vi "NN_Layer_Get_OutRefs_as3D_Tensor.vi"(8 "error in (no error)":errorcluster, 11 "Layer":T1={"Name"="", "Layer_Data"=variant, "Layer_Type"=enum."Input3D", "Dims_In"={"C"=0, "H"=0, "W"=0}, "Layers_In"=variant, "Dims_Out"={"C"=0, "H"=0, "W"=0}, "Layers_Out"=variant, "Metrics"={"Data"=0.0, "Params"=0.0, "Ops"=0.0}, "GPU_Data"=variant, "mBatch"=0, "NN_Device"=enum."CPU", "NNg_hdls"={"cudnn"=0, "cublas"=0, "stream"=0, "curand"=0}, "Train?"=FALSE, "Dimty"=enum."1D", "RecptField"={"Dims"={"V"=0, "H"=0}, "J"={"V"=0, "H"=0}}} {"Metrics"."Data" format="%#_4p"; "Metrics"."Params" format="%#_4p"; "Metrics"."Ops" format="%#_4p"}) -> (0 "error out":errorcluster, 2 "dOut":refnum<class "T4D_SGL.lvclass">, 3 "Out":refnum<class "T4D_SGL.lvclass">)   [LabVIEW 2020]
uses:
  <vilib>/Ngene/Deep Learning Toolkit/Toolkit/NN_Layers/Controls/NN_Layer.ctl
  <vilib>/Ngene/Deep Learning Toolkit/Toolkit/NN_Layers/Controls/NN_Layer_Type.ctl
  <vilib>/Ngene/Deep Learning Toolkit/Toolkit/NN_Data/API/NN_Dims(C,H,W).ctl
  <vilib>/Ngene/Deep Learning Toolkit/Toolkit/NN_Layers/Controls/NN_Layer_Metrics.ctl
  <vilib>/Ngene/Deep Learning Toolkit/Toolkit/NN_Network/Controls/NN_Device.ctl
  <vilib>/Ngene/Deep Learning Toolkit/Toolkit/NNg/cuda/Controls/nng_cuda_handles.ctl
  <vilib>/Ngene/Deep Learning Toolkit/Toolkit/NN_Layers/Controls/NN_Layer_Dimty.ctl
  <vilib>/Ngene/Deep Learning Toolkit/Toolkit/NN_Layers/Controls/NN_Layer_RF_State.ctl
  <vilib>/Ngene/Deep Learning Toolkit/Toolkit/NN_Data/API/NN_Dims(V,H).ctl
  <vilib>/Ngene/CuLab - GPU Accelerated Toolkit/Toolkit/Low_Level/Tensor_Classes/T_Children/T4D/T4D_Children/T4D_SGL/T4D_SGL.lvclass
  <vilib>/Ngene/Deep Learning Toolkit/Toolkit/NN_Layers/Layers/Input/API/NN_Layer_Get_Data(Input3D).vi
  <vilib>/Ngene/Deep Learning Toolkit/Toolkit/NN_Layers/Layers/Activation/API/NN_Layer_Get_Data(Activation).vi
  <vilib>/Ngene/Deep Learning Toolkit/Toolkit/NN_Layers/Layers/BatchNorm/API/NN_Layer_Get_Data(BatchNormalization).vi
  <vilib>/Ngene/Deep Learning Toolkit/Toolkit/NN_Layers/Layers/Conv2D_Adv/API/NN_Layer_Get_Data(Conv2D_Adv).vi
  <vilib>/Ngene/Deep Learning Toolkit/Toolkit/NN_Layers/Layers/Pool/API/NN_Layer_Get_Data(Pool).vi
  <vilib>/Ngene/Deep Learning Toolkit/Toolkit/NN_Layers/Layers/UpSample/API/NN_Layer_Get_Data(UpSample).vi
  <vilib>/Ngene/Deep Learning Toolkit/Toolkit/NN_Layers/Layers/DropOut3D/API/NN_Layer_Get_Data(DropOut3D).vi
  <vilib>/Ngene/Deep Learning Toolkit/Toolkit/NNg/Layers/ShortCut/NN_Layer_Get_Data(ShortCut).vi
  <vilib>/Ngene/Deep Learning Toolkit/Toolkit/NN_Layers/Layers/Concat/API/NN_Layer_Get_Data(Concat).vi
  <vilib>/Ngene/Deep Learning Toolkit/Toolkit/NN_Layers/Layers/SoftMax3D/API/NN_Layer_Get_Data(SoftMax3D).vi
  <vilib>/Ngene/CuLab - GPU Accelerated Toolkit/Toolkit/Low_Level/Tensor_Classes/T_Children/T4D/T4D_Children/T4D_SGL/Push.vi
  <vilib>/Ngene/Deep Learning Toolkit/Toolkit/Deep_Learning_Toolkit_by_Ngene.lvlib
  <vilib>/Ngene/CuLab - GPU Accelerated Toolkit/Toolkit/CuLab.lvlib
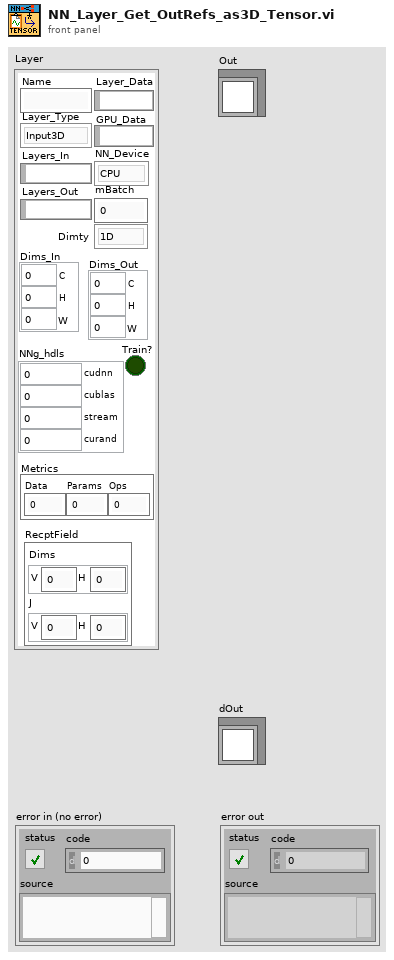
[diagram p1: front panel]
types:
  T1 = typedef "Deep_Learning_Toolkit_by_Ngene.lvlib/NN_Layer.ctl" = cluster{"Name":string, "Layer_Data":variant, "Layer_Type":T2, "Dims_In":T3, "Layers_In":variant, "Dims_Out":T3, "Layers_Out":variant, "Metrics":T4, "GPU_Data":variant, "mBatch":i32, "NN_Device":T5, "NNg_hdls":T6, "Train?":bool, "Dimty":T7, "RecptField":T8}
  T2 = typedef "Deep_Learning_Toolkit_by_Ngene.lvlib/NN_Layer_Type.ctl" = enum16{"Input1D", "Input3D", "Conv1D", "Conv2D", "Conv2D_Adv", "MaxPool", "AvgPool", "UpSample", "DropOut3D", "ShortCut", "Concat", "SoftMax3D", "FC", "DropOut", "Softmax", "Flatten", "YOLO_v2", "YOLO_v4", "Activation", "BatchNormalization", "Unsupported"}
  T3 = typedef "Deep_Learning_Toolkit_by_Ngene.lvlib/NN_Dims(C,H,W).ctl" = cluster{"C":i32, "H":i32, "W":i32}
  T4 = typedef "Deep_Learning_Toolkit_by_Ngene.lvlib/NN_Layer_Metrics.ctl" = cluster{"Data":dbl, "Params":dbl, "Ops":dbl}
  T5 = typedef "Deep_Learning_Toolkit_by_Ngene.lvlib/NN_Device.ctl" = enum16{"CPU", "GPU"}
  T6 = typedef "Deep_Learning_Toolkit_by_Ngene.lvlib/nng_cuda_handles.ctl" = cluster{"cudnn":u64, "cublas":u64, "stream":u64, "curand":u64}
  T7 = typedef "Deep_Learning_Toolkit_by_Ngene.lvlib/NN_Layer_Dimty.ctl" = enum16{"1D", "3D"}
  T8 = typedef "Deep_Learning_Toolkit_by_Ngene.lvlib/NN_Layer_RF_State.ctl" = cluster{"Dims":T9, "J":T9}
  T9 = typedef "Deep_Learning_Toolkit_by_Ngene.lvlib/NN_Dims(V,H).ctl" = cluster{"V":i32, "H":i32}
  T10 = typedef "Deep_Learning_Toolkit_by_Ngene.lvlib/NN_Layer_Data(Input3D).ctl" = cluster{"Out":T11, "Aug Config Params":T12, "WS":variant, "WS_dtype":T16, "Shifts":sgl[], "Scales":sgl[]}
  T11 = typedef "Deep_Learning_Toolkit_by_Ngene.lvlib/NN_Data_ref(4D_SGL).ctl" = refnum<data-value>
  T12 = typedef "Deep_Learning_Toolkit_by_Ngene.lvlib/NN_Layer_Config_Aug(Input3D).ctl" = T13[]
  T13 = typedef "Deep_Learning_Toolkit_by_Ngene.lvlib/NN_Input3D_Aug_Config.ctl" = cluster{"Aug Type":T14, "Aug Value":sgl, "Distribution Type":T15}
  T14 = typedef "Deep_Learning_Toolkit_by_Ngene.lvlib/NN_Input3D_Aug_Types.ctl" = enum16{"Flip_H", "Flip_V", "Brightness", "Contrast", "Noise", "Blur", "Saturation", "Rotate", "Move", "Skew_X", "Skew_Y", "Zoom"}
  T15 = typedef "Deep_Learning_Toolkit_by_Ngene.lvlib/Aug_Distribution_Type.ctl" = enum16{"Uniform", "Gaussian"}
  T16 = typedef "Deep_Learning_Toolkit_by_Ngene.lvlib/NN_Data_type.ctl" = enum16{"I8", "U8", "I16", "U16", "U32 ARGB", "SGL"}
  T17 = typedef "Deep_Learning_Toolkit_by_Ngene.lvlib/NN_Layer_Data(Activation)_3D.ctl" = cluster{"Activation":T18, "Out":T11, "dOut":T11, "Activation_WS":T11}
  T18 = typedef "Deep_Learning_Toolkit_by_Ngene.lvlib/NN_Activation_Type.ctl" = enum16{"Sigmoid", "ReLU", "LReLU", "ReLU6", "tanh", "Swish", "Mish", "None"}
  T19 = typedef "Deep_Learning_Toolkit_by_Ngene.lvlib/NN_Layer_Data(BatchNormalization3D).ctl" = cluster{"Out":T11, "dOut":T11, "BN3D_Data_Refs":T20}
  T20 = typedef "Deep_Learning_Toolkit_by_Ngene.lvlib/NN_BN3D_Data.ctl" = cluster{"scales":T21, "roll_mean":T21, "roll_var":T21, "b":T21, "train":T22, "x":T11, "x_norm":T11, "Adam":T23, "b_Adam":T23, "epsilon":sgl, "expAvgFactor":sgl}
  T21 = typedef "Deep_Learning_Toolkit_by_Ngene.lvlib/NN_Data_ref(1D_SGL).ctl" = refnum<data-value>
  T22 = typedef "Deep_Learning_Toolkit_by_Ngene.lvlib/NN_BN_Train_Data.ctl" = cluster{"dscale":T21, "mean ":T21, "dmean ":T21, "var ":T21, "dvar ":T21, "db":T21}
  T23 = typedef "Deep_Learning_Toolkit_by_Ngene.lvlib/NN_Adam_Weights(1D).ctl" = cluster{"m":T21, "v":T21}
  T24 = typedef "Deep_Learning_Toolkit_by_Ngene.lvlib/NN_Layer_Data(Conv2D_Adv).ctl" = cluster{"W":T25, "b":T21, "Out":T11, "dW":T25, "db":T21, "dOut":T11, "BN":bool, "BN_Data":T20, "WS":T25, "Pool_Type":T26, "Activation":T18, "Conv2D_Advanced_Params":T27, "Activation_WS":T11, "W_Adam":T29, "b_Adam":T23, "Has Bias?":bool}
  T25 = typedef "Deep_Learning_Toolkit_by_Ngene.lvlib/NN_Data_ref(2D_SGL).ctl" = refnum<data-value>
  T26 = typedef "Deep_Learning_Toolkit_by_Ngene.lvlib/NN_Layer_Pool_Type.ctl" = enum16{"None", "Max", "Avg"}
  T27 = typedef "Deep_Learning_Toolkit_by_Ngene.lvlib/NN_Layer_Params(Conv2D_Adv).ctl" = cluster{"Filters":i32, "Groups":i32, "Kernel_Size":T9, "Stride":T9, "Pad_Type":T28, "Pad_Size":T9, "Dilation":T9}
  T28 = typedef "Deep_Learning_Toolkit_by_Ngene.lvlib/NN_Conv2D_Padding_Type.ctl" = enum16{"Pad_Size", "Valid", "Same"}
  T29 = typedef "Deep_Learning_Toolkit_by_Ngene.lvlib/NN_Adam_Weights(2D).ctl" = cluster{"m":T25, "v":T25}
  T30 = typedef "Deep_Learning_Toolkit_by_Ngene.lvlib/NN_Layer_Data(Pool).ctl" = cluster{"Out":T11, "dOut":T11, "idx":T31, "Pool_Params":T32}
  T31 = typedef "Deep_Learning_Toolkit_by_Ngene.lvlib/NN_Data_ref(5D_I32).ctl" = refnum<data-value>
  T32 = typedef "Deep_Learning_Toolkit_by_Ngene.lvlib/NN_Layer_Params(Pool).ctl" = cluster{"Pool_Type":T26, "Size":T9, "Stride":T9, "Pad_Type":T28, "Pad_Size":T9}
  T33 = typedef "Deep_Learning_Toolkit_by_Ngene.lvlib/NN_Layer_Data(UpSample).ctl" = cluster{"Out":T11, "dOut":T11, "UpSample_Params":T34}
  T34 = typedef "Deep_Learning_Toolkit_by_Ngene.lvlib/NN_Layer_Params(UpSample).ctl" = cluster{"Stride":T9}
  T35 = typedef "Deep_Learning_Toolkit_by_Ngene.lvlib/NN_Layer_Data(DropOut3D).ctl" = cluster{"Out":T11, "dOut":T11, "mask":T11, "Scale":sgl, "Probability":sgl}
  T36 = typedef "Deep_Learning_Toolkit_by_Ngene.lvlib/NN_Layer_Data(ShortCut).ctl" = cluster{"Out":T11, "dOut":T11, "Activation_WS":T11, "Activation":T18}
  T37 = typedef "Deep_Learning_Toolkit_by_Ngene.lvlib/NN_Layer_Data(Concat).ctl" = cluster{"Out":T11, "dOut":T11}
  T38 = typedef "Deep_Learning_Toolkit_by_Ngene.lvlib/NN_Layer_Data(SoftMax3D).ctl" = cluster{"Out":T11, "dOut":T11, "SoftMax_Desc_Params":T39}
  T39 = typedef "Deep_Learning_Toolkit_by_Ngene.lvlib/NNg_SoftMax_Desc_Params.ctl" = cluster{"Softmax_Algo":T40, "SoftMax_Mode":T41}
  T40 = typedef "Deep_Learning_Toolkit_by_Ngene.lvlib/cudnnSoftmaxAlgorithm_t.ctl" = enum32{"SOFTMAX_FAST", "SOFTMAX_ACCURATE", "SOFTMAX_LOG"}
  T41 = typedef "Deep_Learning_Toolkit_by_Ngene.lvlib/cudnnSoftmaxMode_t.ctl" = enum32{"Instance", "Channel"}
  T42 = typedef "Deep_Learning_Toolkit_by_Ngene.lvlib/NNg_T4D_Desc.ctl" = cluster{"T4D_desc*":u64, "T4D_Desc":T43, "Size":u64, "gpu_mem":T47}
  T43 = typedef "Deep_Learning_Toolkit_by_Ngene.lvlib/NNg_T4D_Desc_Params.ctl" = cluster{"Format":T44, "Type":T45, "Dims":T46}
  T44 = typedef "Deep_Learning_Toolkit_by_Ngene.lvlib/cudnnTensorFormat_t.ctl" = enum16{"NCHW", "NHWC"}
  T45 = typedef "Deep_Learning_Toolkit_by_Ngene.lvlib/cudnnDataType_t.ctl" = enum16{"FLOAT", "DOUBLE", "HALF", "INT8", "INT32", "INT8x4", "UINT8", "UINT8x4"}
  T46 = typedef "Deep_Learning_Toolkit_by_Ngene.lvlib/NNg_T4D_Dims.ctl" = cluster{"N":i32, "C":i32, "H":i32, "W":i32}
  T47 = typedef "Deep_Learning_Toolkit_by_Ngene.lvlib/cuda_Mem_desc.ctl" = cluster{"Ref*":u64, "Size(B)":u64}
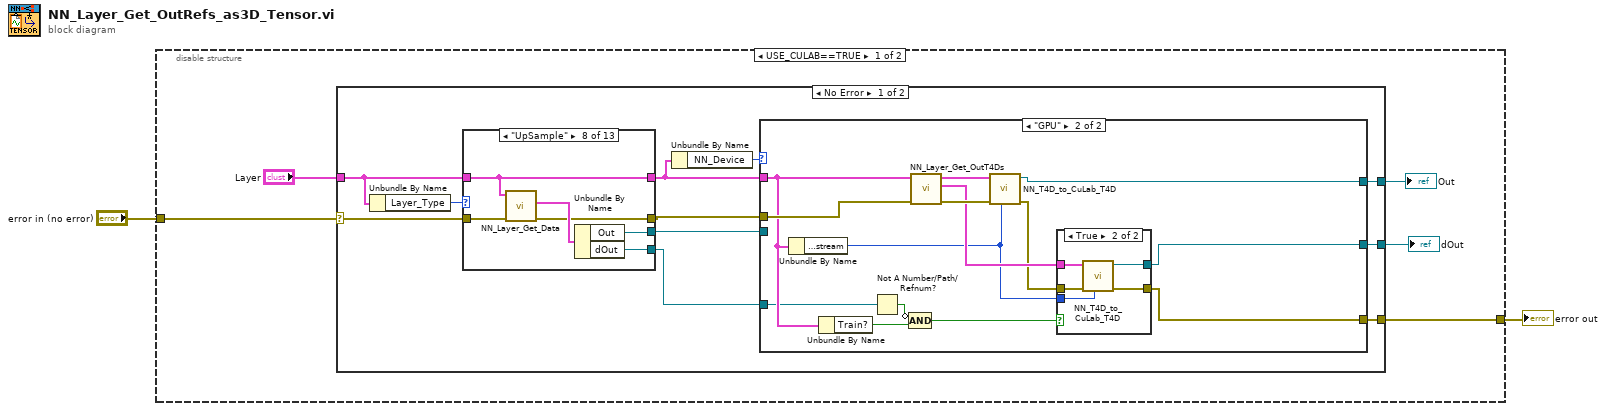
[diagram p0: block diagram]
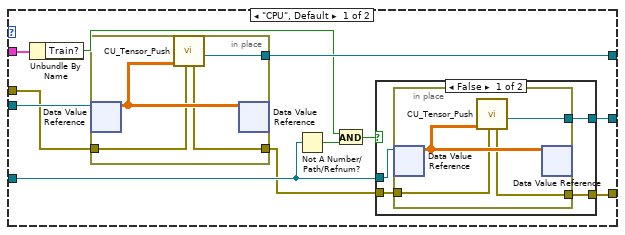
[diagram p2: hidden frame]
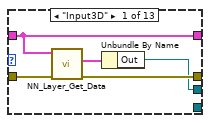
[diagram p5: hidden frame]
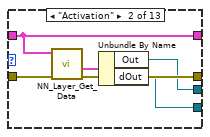
[diagram p6: hidden frame]
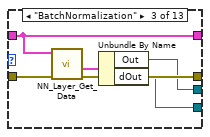
[diagram p7: hidden frame]
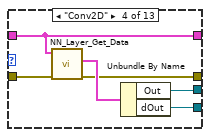
[diagram p8: hidden frame]
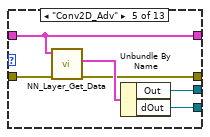
[diagram p9: hidden frame]
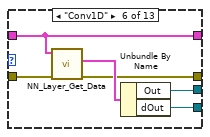
[diagram p10: hidden frame]
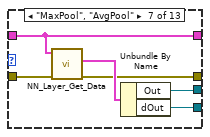
[diagram p11: hidden frame]
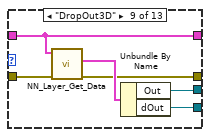
[diagram p12: hidden frame]
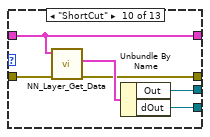
[diagram p13: hidden frame]
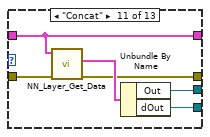
[diagram p14: hidden frame]
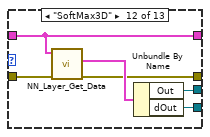
[diagram p15: hidden frame]
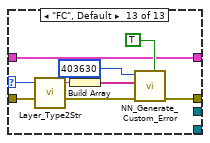
[diagram p16: hidden frame]
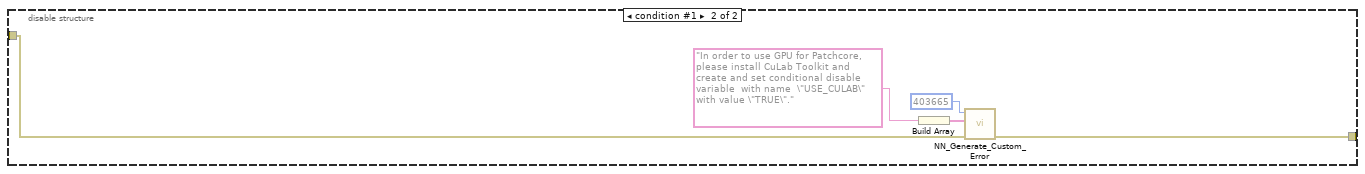
[diagram p18: hidden frame]
diagram:
  n1 = disable-structure shown="USE_CULAB==TRUE" {
    disable-tunnel: "error in (no error)" -> [w4 w144]
    disable-tunnel: [w3 w143] -> w1
    frame condition #0 (active) {
      n2 = case shown="No Error" w4 {
        selector: w4 -> [w8 w142]
        tunnel: "Layer" -> [w17 _]
        tunnel: [w11 _] -> w6
        tunnel: [w10 _] -> w5
        tunnel: [w9 w142] -> w3
        frame No Error {
          n3 = Unbundle By Name(w17) -> ("Layer_Type"=w18:T2)
          n4 = case shown="\"UpSample\"" w18 {
            selector: w18 -> [_ _ _ _ _ _ _ _ _ _ _ _ w137]
            tunnel: w17 -> [w67 w73 w79 w80 w86 w92 w98 w104 w115 w121 w127 w133 w135]
            tunnel: [w66 w72 w78 w83 w89 w95 w101 w107 w112 w118 w124 w130 w138] -> w12
            tunnel: w8 -> [w65 w71 w77 w85 w91 w97 w103 w109 w114 w120 w126 w132 w139]
            tunnel: [_ w68 w74 w81 w87 w93 w99 w105 w110 w116 w122 w128 _] -> w13
            tunnel: [w64 w70 w76 w82 w88 w94 w100 w106 w111 w117 w123 w129 _] -> w14
            tunnel: [w67 w73 w79 w80 w86 w92 w98 w104 w115 w121 w127 w133 w135] -> w15
            frame "Input3D" {
              n5 = call-poly <vilib>:"NN_Layer_Get_Data.vi"("error in (no error)"=w65, "Layer in"=w67) -> ("error out"=w66:errorcluster, "Input3D_Data"=w63:T10)  [unwired: 7 in, 1 out]
              n6 = Unbundle By Name(w63) -> ("Out"=w64:T11)
            }
            frame "Activation" {
              n7 = call-poly <vilib>:"NN_Layer_Get_Data.vi"("error in (no error)"=w71, "Layer in"=w73) -> ("error out"=w72:errorcluster, "Activation_Data_4D"=w69:T17)  [unwired: 6 in, 2 out]
              n8 = Unbundle By Name(w69) -> ("Out"=w70:T11, "dOut"=w68:T11)
            }
            frame "BatchNormalization" {
              n9 = call-poly <vilib>:"NN_Layer_Get_Data.vi"("error in (no error)"=w77, "Layer in"=w79) -> ("error out"=w78:errorcluster, "BN_Data_4D"=w75:T19)  [unwired: 6 in, 2 out]
              n10 = Unbundle By Name(w75) -> ("Out"=w76:T11, "dOut"=w74:T11)
            }
            frame "Conv2D" {
              n11 = call-poly <vilib>:"NN_Layer_Get_Data.vi"("error in (no error)"=w85, "Layer in"=w80) -> ("error out"=w83:errorcluster, "Conv2D_Advanced_Data"=w84:T24)  [unwired: 7 in, 1 out]
              n12 = Unbundle By Name(w84) -> ("Out"=w82:T11, "dOut"=w81:T11)
            }
            frame "Conv2D_Adv" {
              n13 = call-poly <vilib>:"NN_Layer_Get_Data.vi"("error in (no error)"=w91, "Layer in"=w86) -> ("error out"=w89:errorcluster, "Conv2D_Advanced_Data"=w90:T24)  [unwired: 7 in, 1 out]
              n14 = Unbundle By Name(w90) -> ("Out"=w88:T11, "dOut"=w87:T11)
            }
            frame "Conv1D" {
              n15 = call-poly <vilib>:"NN_Layer_Get_Data.vi"("error in (no error)"=w97, "Layer in"=w92) -> ("error out"=w95:errorcluster, "Conv2D_Advanced_Data"=w96:T24)  [unwired: 7 in, 1 out]
              n16 = Unbundle By Name(w96) -> ("Out"=w94:T11, "dOut"=w93:T11)
            }
            frame "MaxPool", "AvgPool" {
              n17 = call-poly <vilib>:"NN_Layer_Get_Data.vi"("error in (no error)"=w103, "Layer in"=w98) -> ("error out"=w101:errorcluster, "Pool_Data"=w102:T30)  [unwired: 7 in, 1 out]
              n18 = Unbundle By Name(w102) -> ("Out"=w100:T11, "dOut"=w99:T11)
            }
            frame "UpSample" {
              n19 = call-poly <vilib>:"NN_Layer_Get_Data.vi"("error in (no error)"=w109, "Layer in"=w104) -> ("error out"=w107:errorcluster, "UpSample_Data"=w108:T33)  [unwired: 7 in, 1 out]
              n20 = Unbundle By Name(w108) -> ("Out"=w106:T11, "dOut"=w105:T11)
            }
            frame "DropOut3D" {
              n21 = call-poly <vilib>:"NN_Layer_Get_Data.vi"("error in (no error)"=w114, "Layer in"=w115) -> ("error out"=w112:errorcluster, "DropOut3D_Data"=w113:T35)  [unwired: 7 in, 1 out]
              n22 = Unbundle By Name(w113) -> ("Out"=w111:T11, "dOut"=w110:T11)
            }
            frame "ShortCut" {
              n23 = call-poly <vilib>:"NN_Layer_Get_Data.vi"("error in (no error)"=w120, "Layer in"=w121) -> ("error out"=w118:errorcluster, "ShortCut_Data"=w119:T36)  [unwired: 7 in, 1 out]
              n24 = Unbundle By Name(w119) -> ("Out"=w117:T11, "dOut"=w116:T11)
            }
            frame "Concat" {
              n25 = call-poly <vilib>:"NN_Layer_Get_Data.vi"("error in (no error)"=w126, "Layer in"=w127) -> ("error out"=w124:errorcluster, "Concat_Data"=w125:T37)  [unwired: 7 in, 1 out]
              n26 = Unbundle By Name(w125) -> ("Out"=w123:T11, "dOut"=w122:T11)
            }
            frame "SoftMax3D" {
              n27 = call-poly <vilib>:"NN_Layer_Get_Data.vi"("error in (no error)"=w132, "Layer in"=w133) -> ("error out"=w130:errorcluster, "SoftMax3D"=w131:T38)  [unwired: 7 in, 1 out]
              n28 = Unbundle By Name(w131) -> ("Out"=w129:T11, "dOut"=w128:T11)
            }
            frame "FC", Default {
              n29 = call <vilib>:"Layer_Type2Str.vi"("Layer_Type"=w137) -> ("Str"=w136:string)  [unwired: 8 in]
              n30 = Build Array(w136) -> (w134:string[])
              n31 = call <vilib>:"NN_Generate_Custom_Error.vi"("show call chain? (False)"=TRUE, "error in (no error)"=w139, "Message"=w134, "Error_code"=403630 ("error code (0)")) -> ("error out"=w138:errorcluster)  [unwired: 7 in]
            }
          }
          n32 = Unbundle By Name(w15) -> ("NN_Device"=w16:T5)
          n33 = case shown="\"GPU\"" w16 {
            tunnel: w15 -> [w21 w54]
            tunnel: [w27 w50] -> w11
            tunnel: [w22 w43] -> w9
            tunnel: w14 -> [w29 _]
            tunnel: [w26 w45] -> w10
            tunnel: w13 -> [w25 w53]
            tunnel: w12 -> [w28 w56]
            frame "CPU", Default {
              n34 = Unbundle By Name(w21) -> ("Train?"=w19:bool)
              n35 = in-place {
                in-place-border: w28 -> [w41]
                in-place-border: [w40] -> w23
                in-place-border: [w39] -> w27
                n36 = in-place-dvr #1(w29) -> (w42:sgl[][][][])  [unwired: 1 out]
                n37 = call-poly <vilib>:"CU_Tensor_Push.vi"("error in (no error)"=w41, "CPU_Data_4D_SGL"=w42) -> ("T4D_SGL out"=w39:refnum<class "T4D_SGL.lvclass">, "error out"=w40:errorcluster)  [unwired: 8 in]
                n38 = in-place-dvr #1(w42) -> ()  [unwired: 2 out]
              }
              n39 = Not A Number/Path/Refnum?(number/path/refnum=w25) -> (NaN/Path/Refnum?=w24:bool)
              n40 = And(x=w19, y=w24) -> (x .and. y?=w20:bool)
              n41 = case shown="False" w20 {
                tunnel: [w33 _] -> w26
                tunnel: w25 -> [w32 _]
                tunnel: w23 -> [w31 w38]
                tunnel: [w30 w38] -> w22
                frame False {
                  n42 = in-place {
                    in-place-border: w31 -> [w36]
                    in-place-border: [w35] -> w30
                    in-place-border: [w34] -> w33
                    n43 = in-place-dvr #2(w32) -> (w37:sgl[][][][])  [unwired: 1 out]
                    n44 = call-poly <vilib>:"CU_Tensor_Push.vi"("error in (no error)"=w36, "CPU_Data_4D_SGL"=w37) -> ("T4D_SGL out"=w34:refnum<class "T4D_SGL.lvclass">, "error out"=w35:errorcluster)  [unwired: 8 in]
                    n45 = in-place-dvr #2(w37) -> ()  [unwired: 2 out]
                  }
                }
                frame True {
                }
              }
            }
            frame "GPU" {
              n46 = Unbundle By Name(w54) -> ("NNg_hdls.stream"=w44:u64)
              n47 = Unbundle By Name(w54) -> ("Train?"=w55:bool)
              n48 = Not A Number/Path/Refnum?(number/path/refnum=w53) -> (NaN/Path/Refnum?=w52:bool)
              n49 = Compound Arithmetic op=AND(invert w52, w55) -> (w48:bool)
              n50 = call <vilib>:"NN_Layer_Get_OutT4Ds.vi"("error in"=w56, "Layer in"=w54) -> ("error out"=w51:errorcluster, "T4D_dOut"=w47:T42, "T4D_Out"=w49:T42)  [unwired: 7 in]
              n51 = call "NN_T4D_to_CuLab_T4D.vi"("stream"=w44, "error in (no error)"=w51, "T4D_Out"=w49) -> ("error out"=w46:errorcluster, "T4D_SGL out"=w50:refnum<class "T4D_SGL.lvclass">)  [unwired: 7 in]
              n52 = case shown="True" w48 {
                tunnel: w47 -> [_ w62]
                tunnel: w46 -> [w57 w61]
                tunnel: [_ w60] -> w45
                tunnel: w44 -> [_ w59]
                tunnel: [w57 w58] -> w43
                frame False {
                }
                frame True {
                  n53 = call "NN_T4D_to_CuLab_T4D.vi"("stream"=w59, "error in (no error)"=w61, "T4D_Out"=w62) -> ("error out"=w58:errorcluster, "T4D_SGL out"=w60:refnum<class "T4D_SGL.lvclass">)  [unwired: 7 in]
                }
              }
            }
          }
        }
        frame Error {
        }
      }
      "dOut" <- w5
      "Out" <- w6
    }
    frame condition #1 {
      n54 = Build Array("In order to use GPU for Patchcore, please install CuLab Toolkit and create and set conditional disable variable  with name  \"USE_CULAB\" with value \"TRUE\"." ("Message")) -> (w146:string[])
      n55 = call <vilib>:"NN_Generate_Custom_Error.vi"("error in (no error)"=w144, "Message"=w146, "Error_code"=403665) -> ("error out"=w143:errorcluster)  [unwired: 8 in]
    }
  }
  "error out" <- w1
